vi "Call.vi"(8 "error in (no error)":errorcluster, 9 "Inputs":variant, 10 "Method Name":string, 11 "SMOFacade in":refnum<class "SMOFacade.lvclass">) -> (0 "error out":errorcluster, 1 "Outputs":variant, 2 "Method Name dup":string, 3 "SMOFacade out":refnum<class "SMOFacade.lvclass">)   [LabVIEW 2013, in "SMOFacade.lvclass"]
uses:
  SMOFacade.lvclass
  Registry/SMO_API--Cluster.ctl
  Control Definition -- Cluster.ctl
  <vilib>/Utility/VariantDataType/Type.ctl
  SMOFacade.lvclass/SMOFacade.ctl
  Registry/Registry-SMO.lvclass
  <vilib>/Utility/VariantDataType/VariantType.lvlib
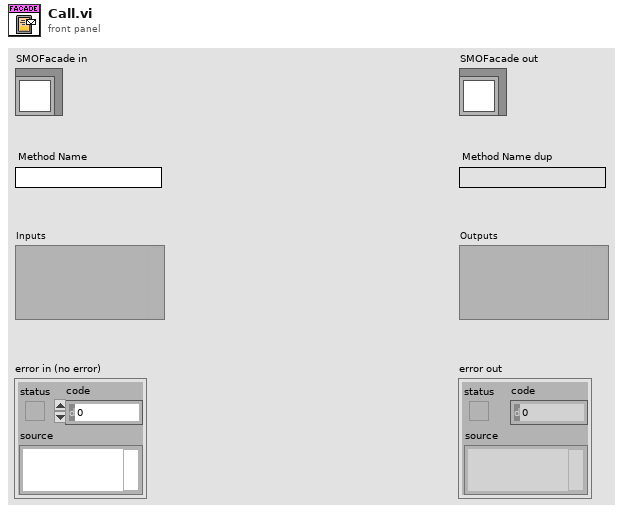
[diagram p1: front panel]
types:
  T1 = typedef "Registry-SMO.lvclass/SMO_API--Cluster.ctl" = cluster{"Method Name":string, "Full Method Name":string, "input string":string, "output string":string, "input type":variant, "output type":variant, "prototype":string, "Inputs":T2[], "Outputs":T2[], "SMO Input":T2, "Error Output":T2}
  T2 = typedef "Registry-SMO.lvclass/Control Definition -- Cluster.ctl" = cluster{"Type Enum":T3, "Caption.Text":string, "DefVal":variant, "ControlIndex":i32, "Label.Text":string, "Required":bool, "SMO Input":bool, "Error Output":bool}
  T3 = typedef "VariantType.lvlib/Type.ctl" = enum8{"Invalid Type", "Void", "I8", "I16", "I32", "I64", "U8", "U16", "U32", "U64", "Single Float", "Double Float", "Extended Float", "Single Complex", "Double Complex", "Extended Complex", "Enum U8", "Enum U16", "Enum U32", "Enum U64", "Single Float With Unit", "Double Float With Unit", "Extended Float With Unit", "Single Complex with Unit", "Double Complex with Unit", "Extended Complex with Unit", "Boolean", "String", "Path", "Picture", "Tag", "Array", "Cluster", "Variant", "LV Variant", "Waveform", "Timestamp", "Digital Waveform", "Digital Data", "ExpressData", "Refnum", "External Data", "VI", "Poly VI", "LabVIEW Class Instance", "Fixed Point"}
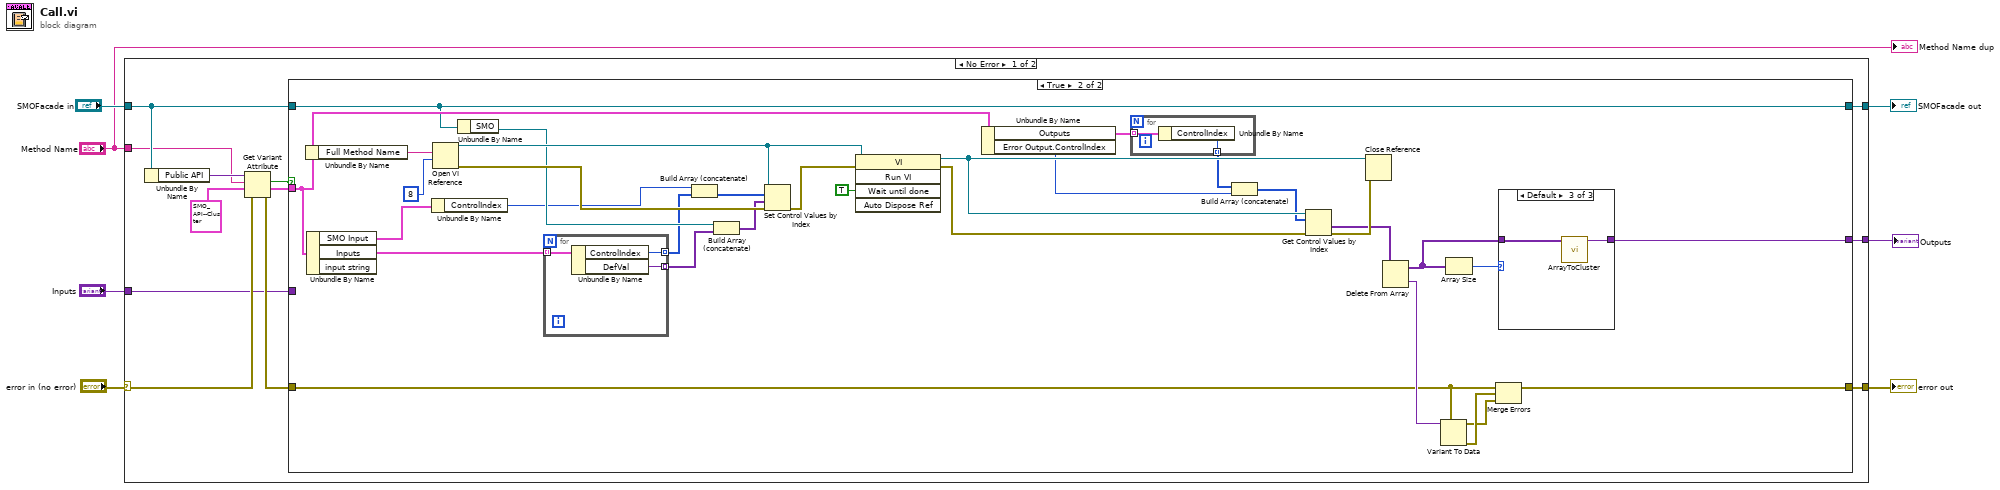
[diagram p0: block diagram]
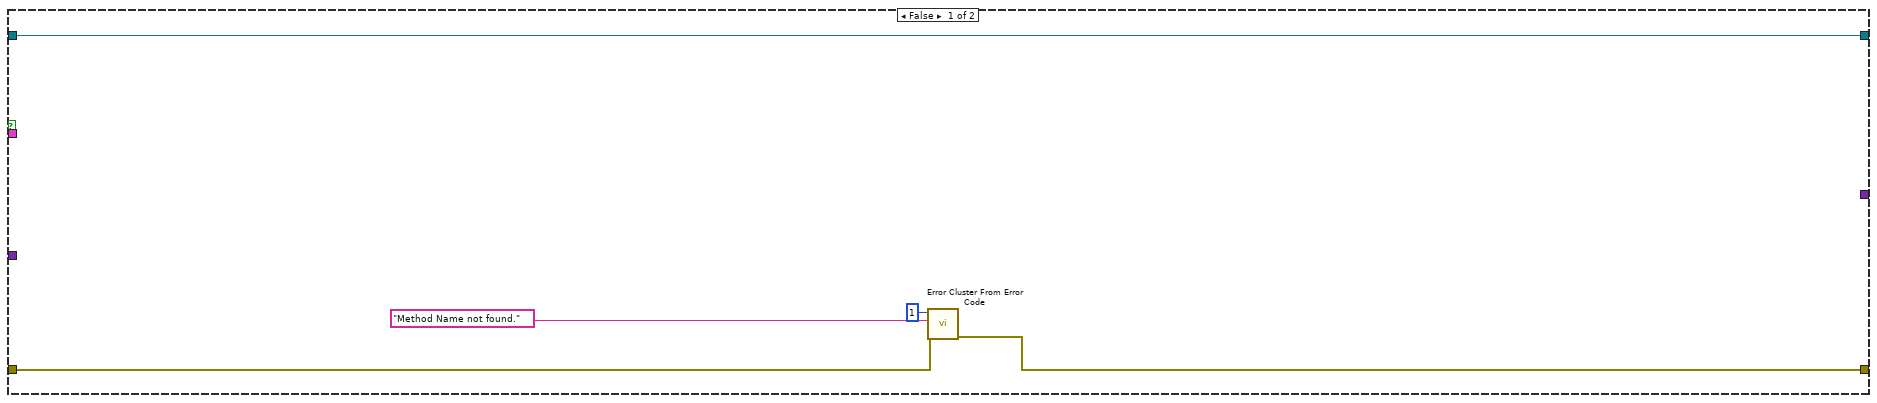
[diagram p2: hidden frame]
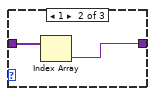
[diagram p4: hidden frame]
diagram:
  n1 = case shown="No Error" "error in (no error)" {
    selector: "error in (no error)" -> [w15 w66]
    tunnel: "SMOFacade in" -> [w19 w67]
    tunnel: [w13 w67] -> w6
    tunnel: "Method Name" -> [w17 _]
    tunnel: [w11 w66] -> w4
    tunnel: "Inputs" -> [w9 _]
    tunnel: [w8 _] -> w1
    frame No Error {
      n2 = Unbundle By Name(w19) -> ("Public API"=w18:variant)
      n3 = Get Variant Attribute(Variant=w18, name=w17, default value (empty Variant)=T1 {"Method Name"="", "Full Method Name"="", "input string"="", "output string"="", "input type"=variant, "output type"=variant, "prototype"="", "Inputs"=[], "Outputs"=[], "SMO Input"={"Type Enum"=enum."Invalid Type", "Caption.Text"="", "DefVal"=variant, "ControlIndex"=0, "Label.Text"="", "Required"=FALSE, "SMO Input"=FALSE, "Error Output"=FALSE}, "Error Output"={"Type Enum"=enum."Invalid Type", "Caption.Text"="", "DefVal"=variant, "ControlIndex"=0, "Label.Text"="", "Required"=FALSE, "SMO Input"=FALSE, "Error Output"=FALSE}} ("API"), error in=w15) -> (found=w14:bool, value=w10:T1, error out=w12:errorcluster)  [unwired: 1 out]
      n4 = case shown="True" w14 {
        tunnel: w19 -> [w24 w42]
        tunnel: [w24 w42] -> w13
        tunnel: w12 -> [w23 w25]
        tunnel: [w22 w27] -> w11
        tunnel: w10 -> [_ w48]
        tunnel: w9 -> [_ _]
        tunnel: [_ w54] -> w8
        frame False {
          n5 = call <vilib>:"Error Cluster From Error Code.vi"("error in (no error)"=w23, "error message (\"\")"="Method Name not found.", "error code (0)"=1) -> ("error out"=w22:errorcluster)  [unwired: 6 in]
        }
        frame True {
          n6 = Unbundle By Name(w48) -> ("Full Method Name"=w52:string)
          n7 = Unbundle By Name(w48) -> ("SMO Input"=w36:T2, "Inputs"=w53:T2[])  [unwired: 1 out]
          n8 = Unbundle By Name(w36) -> ("ControlIndex"=w35:i32)
          n9 = Open VI Reference(vi path=w52, options=8) -> (vi reference=w50:refnum<vi>, error out=w51:errorcluster)  [unwired: 4 in]
          n10 = Unbundle By Name(w42) -> ("SMO"=w41:refnum<class "SMO.lvclass">)
          n11 = for {
            tunnel: w53 -> [w59] mode=indexing
            tunnel: [w58] -> w37 mode=indexing
            tunnel: [w57] -> w38 mode=indexing
            n12 = Unbundle By Name(w59) -> ("ControlIndex"=w58:i32, "DefVal"=w57:variant)
          }
          n13 = Build Array (concatenate)(w35, w37) -> (w40:i32[])
          n14 = Build Array (concatenate)(w41, w38) -> (w39:variant[])
          n15 = Set Control Values by Index(0:w50, 1:w40, 2:w39, 3:w51) -> (11:w49:errorcluster)
          n16 = invoke class="VI" method="Run VI"(reference=w50, error in=w49, "Wait until done"=TRUE ("Wait Until Done")) -> (reference out=w45:refnum<vi>, error out=w46:errorcluster)  [unwired: 2 in, 3 out]
          n17 = Unbundle By Name(w48) -> ("Outputs"=w47:T2[], "Error Output.ControlIndex"=w34:i32)
          n18 = for {
            tunnel: w47 -> [w61] mode=indexing
            tunnel: [w60] -> w32 mode=indexing
            n19 = Unbundle By Name(w61) -> ("ControlIndex"=w60:i32)
          }
          n20 = Build Array (concatenate)(w32, w34) -> (w33:i32[])
          n21 = Get Control Values by Index(0:w45, 1:w33, 3:w46) -> (10:w31:variant[], 11:w44:errorcluster)
          n22 = Close Reference(reference=w45, error in (no error)=w44) -> ()  [unwired: 1 out]
          n23 = Delete From Array(array=w31) -> (deleted portion=w29:variant, array with subset deleted=w30:variant[])  [unwired: 2 in]
          n24 = Variant To Data(type=w25, Variant=w29) -> (data=w26:errorcluster, error out=w28:errorcluster)  [unwired: 1 in]
          n25 = Array Size(array=w30) -> (size(s)=w55:i32)
          n26 = Merge Errors(w25, w28, w26) -> (w27:errorcluster)
          n27 = case shown="Default" w55 {
            tunnel: w30 -> [_ w63 w65]
            tunnel: [_ w62 w64] -> w54
            frame 0 {
            }
            frame 1 {
              n28 = Index Array(array=w63) -> (element=w62:variant)  [unwired: 1 in]
            }
            frame Default {
              n29 = call "ArrayToCluster.vi"("Array"=w65) -> ("Cluster"=w64:variant)  [unwired: 10 in]
            }
          }
        }
      }
    }
    frame Error {
    }
  }
  "error out" <- w4
  "SMOFacade out" <- w6
  "Outputs" <- w1
  "Method Name dup" <- "Method Name"
